vi "Hello World.vi"(8 "error in (no error)":errorcluster, 10 "message":string="Hello World ") -> (0 "error out":errorcluster)   [LabVIEW 2017]
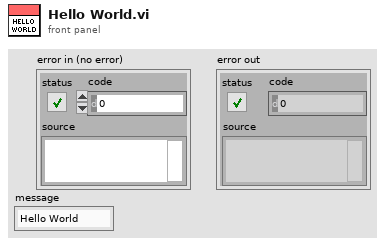
[diagram p1: front panel]
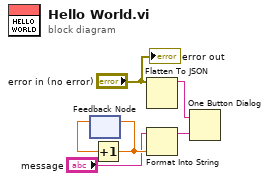
[diagram p0: block diagram]
diagram:
  n1 = feedback #1() -> (w6:dbl)  [unwired: 1 in]
  n2 = Increment(x=w6) -> (x+1=w5:dbl)
  n3 = feedback-in #1(w5) -> ()
  n4 = Flatten To JSON(anything="error in (no error)") -> (JSON string=w1:string)  [unwired: 2 in, 1 out]
  n5 = Format Into String(initial string="message", w5) -> (resulting string=w4:string)  [unwired: 2 in, 1 out]
  n6 = One Button Dialog(message=w1, button name ("OK")=w4) -> ()  [unwired: 1 out]
  "error out" <- "error in (no error)"
